vi "Mdb conn.vi"(1 "input 1":path=path "E:/exam/data/data.mdb") -> (0 "resulting string":string="DBQ=E:\\exam\\data\\data.mdb;DefaultDir=E:\\exam\\data;Driver={Driver do Microsoft Access (*.mdb)};DriverId=25;FIL=MS Access;MaxBufferSize=2048;MaxScanRows=8;PageTimeout=5;SafeTransactions=0;Threads=3;UID=admin;UserCommitSync=Yes;")   [LabVIEW 2010]
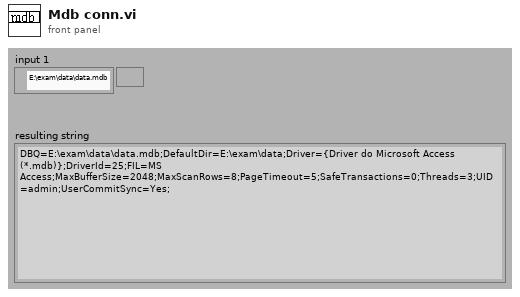
[diagram p1: front panel]
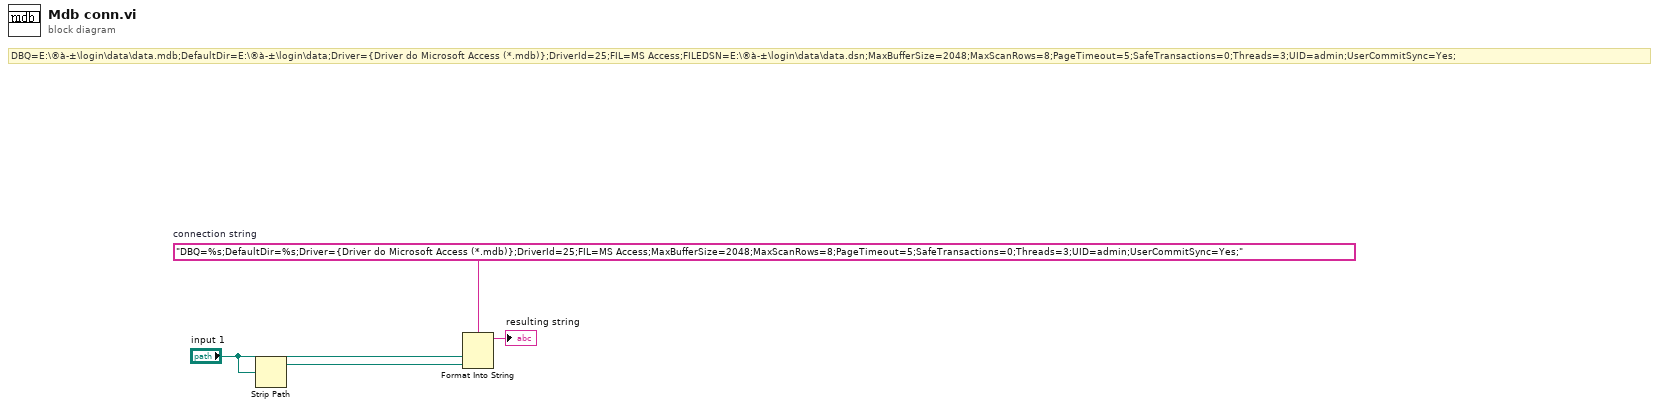
[diagram p0: block diagram]
diagram:
  w3 = "DBQ=%s;DefaultDir=%s;Driver={Driver do Microsoft Access (*.mdb)};DriverId=25;FIL=MS Access;MaxBufferSize=2048;MaxScanRows=8;PageTimeout=5;SafeTransactions=0;Threads=3;UID=admin;UserCommitSync=Yes;"  # connection string
  # "DBQ=E:\\®à­±\\login\\data\\data.mdb;DefaultDir=E:\\®à­±\\login\\data;Driver={Driver do Microsoft Access (*.mdb)};DriverId=25;FIL=MS Access;FILEDSN=E:\\®à­±\\login\\data\\data.dsn;MaxBufferSize=2048;MaxScanRows=8;PageTimeout=5;SafeTransactions=0;Threads=3;UID=admin;UserCommitSync=Yes;"
  n1 = Strip Path(path="input 1") -> (stripped path=w1:path)  [unwired: 1 out]
  n2 = Format Into String(format string=w3, "input 1", w1) -> (resulting string=→"resulting string":string)  [unwired: 2 in, 1 out]
